vi "Constructor.vi"(8 "error in":errorcluster, 10 "FullName":string, 11 "Name":string) -> (0 "error out":errorcluster, 3 "Document out":refnum<class "Characteristic.lvclass">)   [LabVIEW 2021, in "ProligentXMLGenerator.lvlib" / "Characteristic.lvclass"]
uses:
  Characteristic.lvclass
  Characteristic.lvclass/Characteristic.ctl
  Data.ctl
  CustomData/CustomData.lvclass
  Base/NonEmptyString_434/NonEmptyString_434.lvclass
  Base/String_2000/String_2000.lvclass
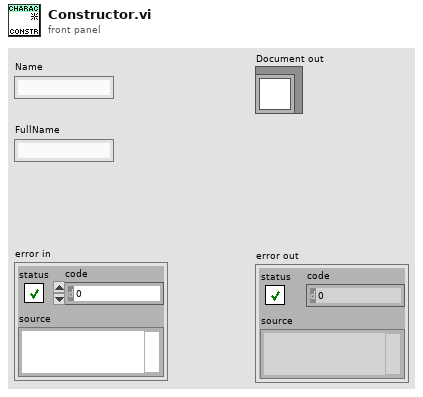
[diagram p1: front panel]
types:
  T1 = typedef "ProligentXMLGenerator.lvlib/Characteristic.lvclass/Data.ctl" = cluster{"Name":string, "CustomData":refnum<class "CustomData.lvclass">, "FullName":refnum<class "NonEmptyString_434.lvclass">, "Value":refnum<class "String_2000.lvclass">}
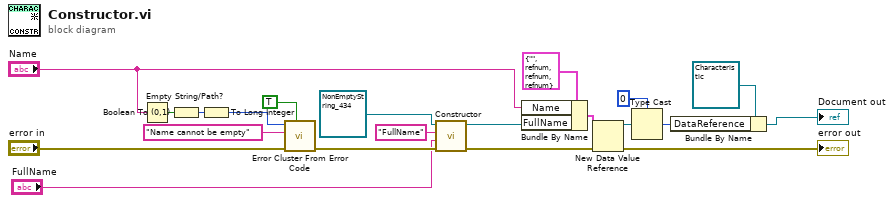
[diagram p0: block diagram]
diagram:
  n1 = Empty String/Path?(string/path="Name") -> (empty?=w12:bool)
  n2 = Boolean To (0,1)(Boolean=w12) -> (0, 1=w11:i16)
  n3 = To Long Integer(number=w11) -> (32bit integer=w10:i32)
  n4 = call <vilib>:"Error Cluster From Error Code.vi"("show call chain? (False)"=TRUE, "error in (no error)"="error in", "error message (\"\")"="Name cannot be empty" ("error message (\"\")"), "error code (0)"=w10) -> ("error out"=w5:errorcluster)  [unwired: 5 in]
  n5 = call-dynamic "Constructor.vi"("error in"=w5, "Value"="FullName", "Name"="FullName", "String in"=refnum<class "NonEmptyString_434.lvclass"> refnum ("ProligentResultProcessor:NonEmptyString_434")) -> ("error out"=w1:errorcluster, "String out"=w2:refnum<class "NonEmptyString_434.lvclass">)  [unwired: 6 in]
  n6 = Bundle By Name(cluster=T1 {"Name"="", "CustomData"=refnum, "FullName"=refnum, "Value"=refnum} ("Data"), "Name"="Name", "FullName"=w2) -> (w17:T1)
  n7 = New Data Value Reference(data value=w17, error in=w1) -> (data value reference=w16:refnum<data-value>, error out=→"error out":errorcluster)
  n8 = Type Cast(type=u64 0, x=w16) -> (*(type *) &x=w14:u64)
  n9 = Bundle By Name(cluster=refnum<class "Characteristic.lvclass"> refnum ("ProligentResultProcessor:CustomData"), "DataReference"=w14) -> (→"Document out":refnum<class "Characteristic.lvclass">)
